vi "Write timed out.vi"(8 "error in (no error)":errorcluster, 10 "timed out?":bool, 11 "Dialog.lvclass in":refnum<class "Dialog.lvclass">) -> (0 "error out":errorcluster, 3 "Dialog.lvclass out":refnum<class "Dialog.lvclass">)   [LabVIEW 2012, in "Dialog.lvlib" / "Dialog.lvclass"]
doc: "Accessor VI for Dialog class."
uses:
  Dialog.lvclass
  Dialog.lvclass/Dialog.ctl
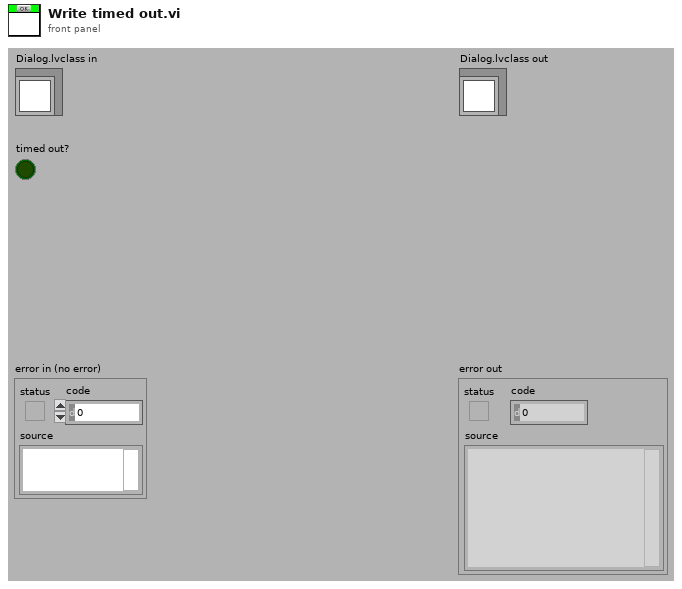
[diagram p1: front panel]
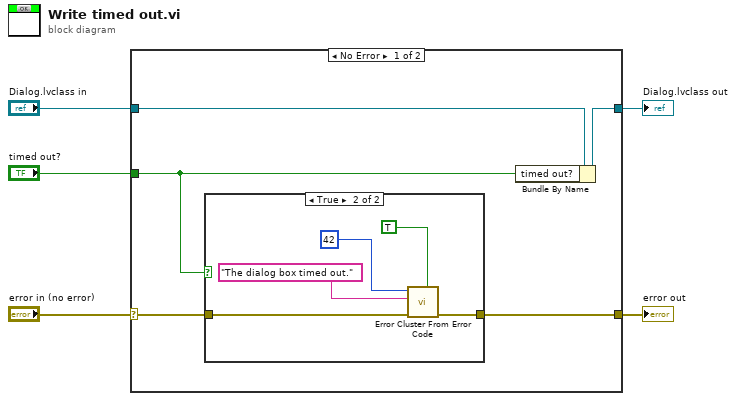
[diagram p0: block diagram]
diagram:
  n1 = case shown="No Error" "error in (no error)" {
    selector: "error in (no error)" -> [w7 w17]
    tunnel: [w8 w17] -> w4
    tunnel: [w9 w18] -> w2
    tunnel: "Dialog.lvclass in" -> [w10 w18]
    tunnel: "timed out?" -> [w6 _]
    frame No Error {
      n2 = case shown="True" w6 {
        tunnel: [w11 w15] -> w8
        tunnel: w7 -> [w11 w14]
        frame False {
        }
        frame True {
          n3 = call <vilib>:"Error Cluster From Error Code.vi"("is warning? (False)"=TRUE, "error in (no error)"=w14, "error message (\"\")"="The dialog box timed out." ("error message (\"\")"), "error code (0)"=42) -> ("error out"=w15:errorcluster)  [unwired: 1 in, 4 out]
        }
      }
      n4 = Bundle By Name(cluster=w10, "timed out?"=w6) -> (w9:refnum<class "Dialog.lvclass">)
    }
    frame Error {
    }
  }
  "error out" <- w4
  "Dialog.lvclass out" <- w2
